vi "Device Scan SubVI.vi"(7 "Simulated Data":bool, 11 "error in (no error)":errorcluster) -> (3 "return count":u32, 4 "VISA INSTRUMENT 1":refnum<visa-resource-name>, 6 "VISA INSTRUMENT 2":refnum<visa-resource-name>, 8 "find list":string[](array[string]), 10 "Terminate":bool, 15 "error out":errorcluster)   [LabVIEW 2017]
uses:
  <vilib>/Instr/_visa.llb/VISA Find Search Mode.ctl
panel:
  # "This VI identifies the GPIB equipment attached to this computer, and searches to see it the following equipment\nis attached:\n\n(1)ASRL1::INSTR - Serial connection port between chromalox controller and computer\n(2)ASRL10::INSTR - Parallel connection port between elevator relays and computer"
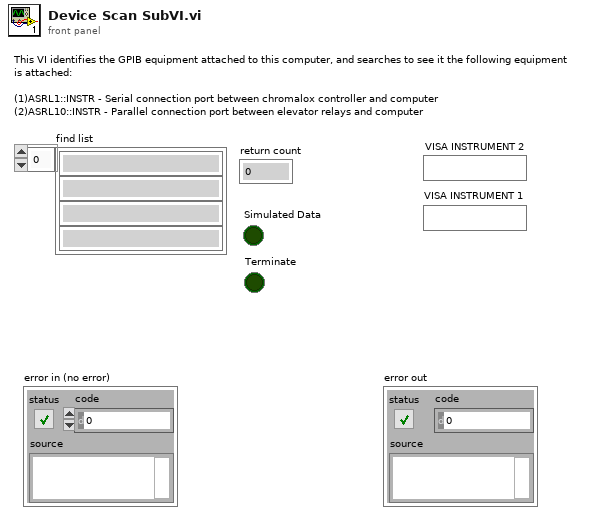
[diagram p1: front panel]
types:
  T1 = typedef "VISA Find Search Mode.ctl" = u32
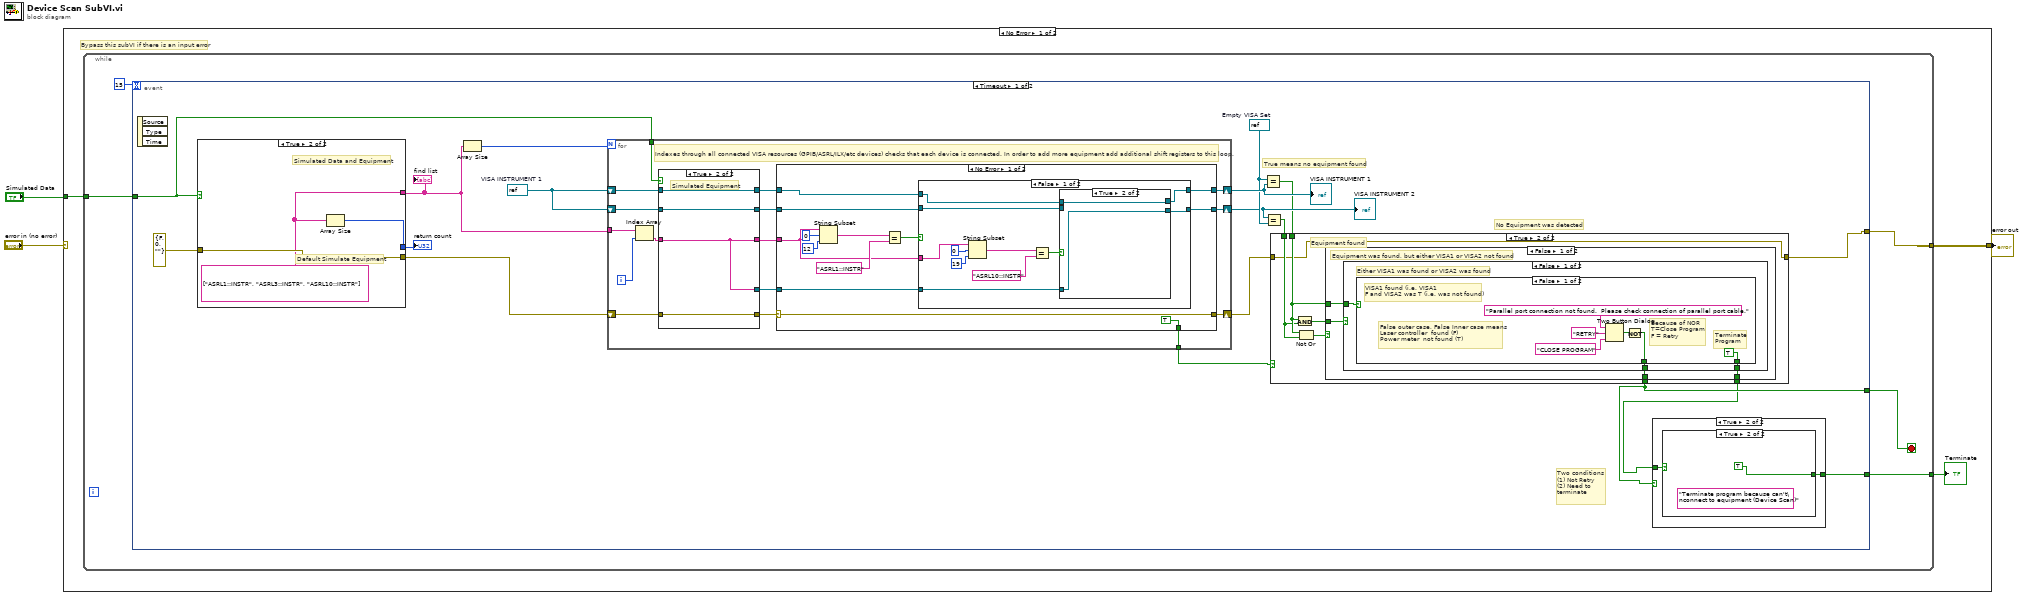
[diagram p0: block diagram]
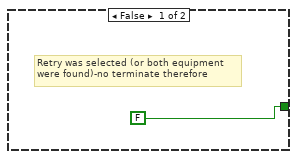
[diagram p2: hidden frame]
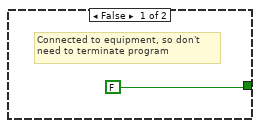
[diagram p3: hidden frame]
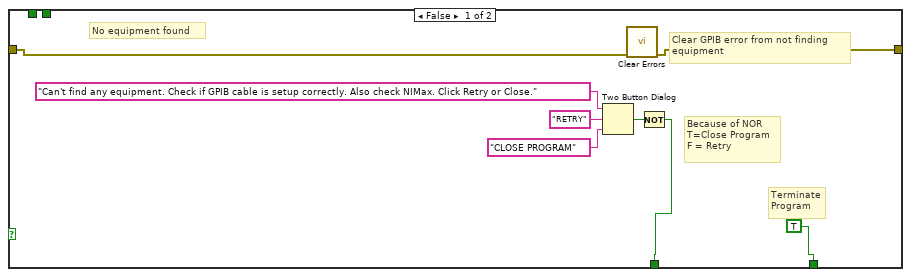
[diagram p4: hidden frame]
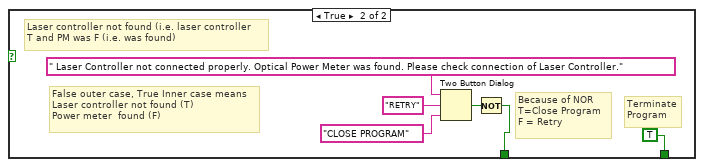
[diagram p5: hidden frame]
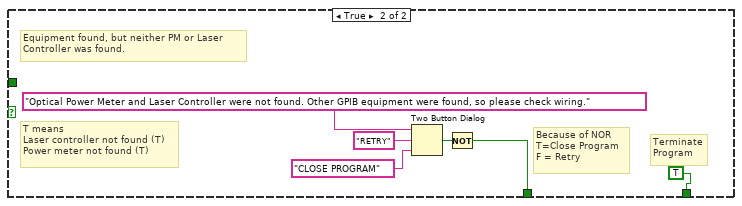
[diagram p6: hidden frame]
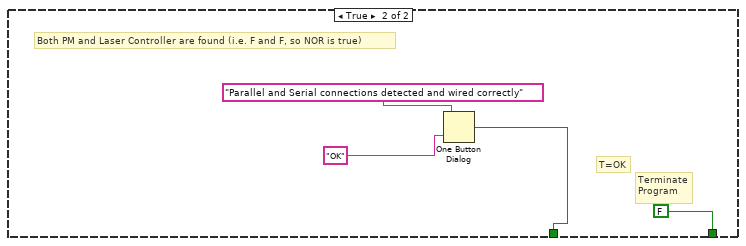
[diagram p7: hidden frame]
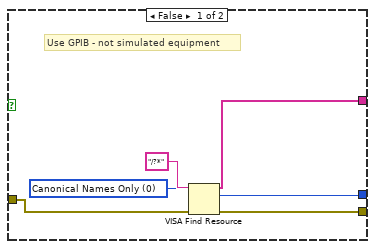
[diagram p8: hidden frame]
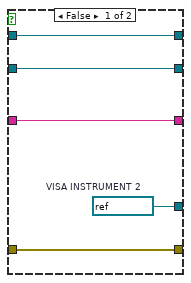
[diagram p9: hidden frame]
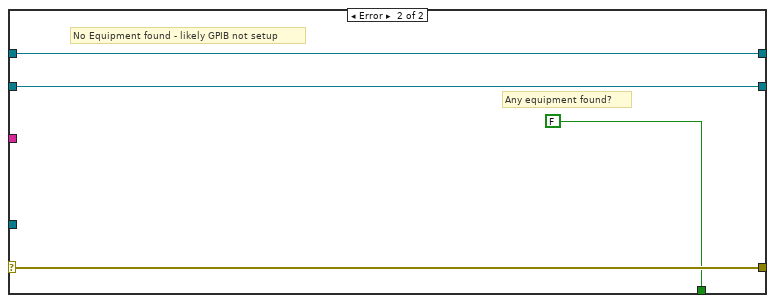
[diagram p12: hidden frame]
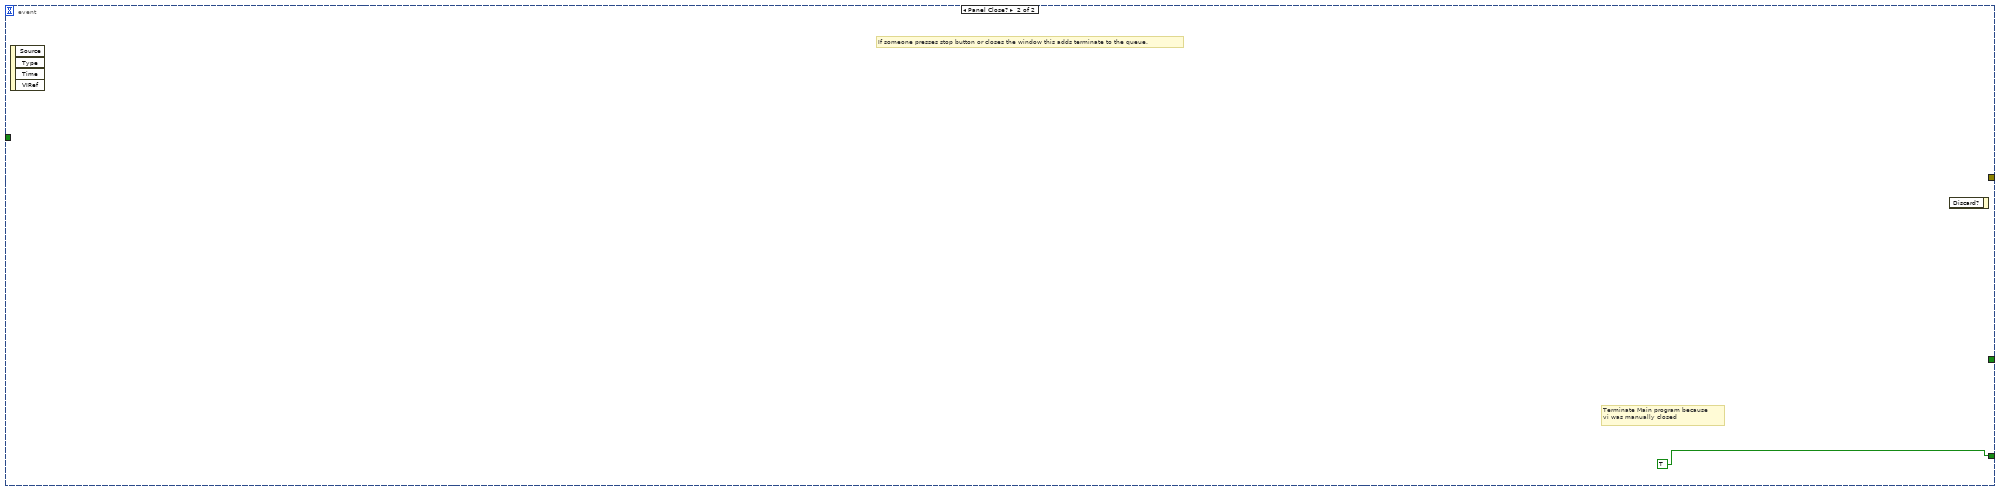
[diagram p13: hidden frame]
diagram:
  n1 = case shown="No Error" "error in (no error)" {
    selector: "error in (no error)" -> [_ w148]
    tunnel: [w6 w148] -> w2
    tunnel: "Simulated Data" -> [w5 _]
    frame No Error {
      # "Bypass this subVI if there is an input error"
      n2 = while {
        tunnel: [w10] -> w6
        tunnel: w5 -> [w9]
        tunnel: [w7] -> w4
        stop <- w11 stop-if-true
        n3 = event shown="[0] Timeout" {
          selector: _ -> [_ _]
          dyn-events: _ -> [_ _]
          timeout: 15 -> [_ _]
          tunnel: [w17 _] -> w11
          tunnel: [w13 _] -> w10
          tunnel: w9 -> [w21 _]
          tunnel: [w15 TRUE] -> w7
          event Timeout {
            w23 = refnum<visa-resource-name> refnum  # Empty VISA Set
            w12 = refnum<visa-resource-name> refnum  # VISA INSTRUMENT 1
            # "Two conditions\n(1) Not Retry\n(2) Need to\nterminate"
            # "No Equipment was detected"
            # "True means no equipment found"
            n4 = event-data() -> ()  [unwired: 1 in, 3 out]
            n5 = case shown="True" w21 {
              tunnel: [w84 w86] -> w28
              tunnel: [w81 w85] -> w27
              tunnel: [w80 w87] -> w26
              tunnel: errorcluster {"status"=FALSE, "code"=0, "source"=""} ("error in (no error) 2") -> [w79 w87]
              frame False {
                w82 = T1 0 items=["Canonical Names Only"=0, "Aliases Only"=2, "Include Matching Aliases"=3, "Include All Aliases"=4] ("Search Mode")
                # "Use GPIB - not simulated equipment"
                n6 = VISA Find Resource(8:w79, 10:w82, 11:"/?*" ("expression (\"?*\")")) -> (0:w80:errorcluster, 2:w84:u32, 3:w81:string[])
              }
              frame True {
                w85 = string[] ["ASRL1::INSTR", "ASRL3::INSTR", "ASRL10::INSTR"] ("Simulated Equipment List")
                # "Default Simulate Equipment"
                # "Simulated Data and Equipment"
                n7 = Array Size(array=w85) -> (size(s)=w86:i32)
              }
            }
            "find list" <- w27
            "return count" <- w28
            n8 = Array Size(array=w27) -> (size(s)=w29:i32)
            n9 = for {
              N: w29 -> [_]
              tunnel: w27 -> [w102]
              shift-right: [w97] -> w22
              shift-left: w12 -> [w93]
              shift-right: [w98] -> w24
              shift-left: w12 -> [w94]
              shift-right: [w95] -> w14
              shift-left: w26 -> [w99]
              tunnel: [w89] -> w18
              tunnel: w21 -> [w90]
              i -> [w103]
              # "Indexes through all connected VISA resources (GPIB/ASRL/ILX/etc devices) checks that each device is connected. In order to add more equipment add additional shift registers to this loop."
              n10 = Index Array(array=w102, index=w103) -> (element=w96:string)
              n11 = case shown="True" w90 {
                tunnel: [w106 w110] -> w101
                tunnel: [w105 w109] -> w100
                tunnel: w99 -> [w106 w110]
                tunnel: w96 -> [w105 w109]
                tunnel: w94 -> [w108 w112]
                tunnel: w93 -> [w107 w111]
                tunnel: [w108 w112] -> w92
                tunnel: [w107 w111] -> w91
                tunnel: [w104 w109] -> w88
                frame False {
                  w104 = refnum<visa-resource-name> refnum  # VISA INSTRUMENT 2
                }
                frame True {
                  # "Simulated Equipment"
                }
              }
              n12 = case shown="No Error" w101 {
                selector: w101 -> [w121 w146]
                tunnel: w100 -> [w117 _]
                tunnel: [w114 w143] -> w97
                tunnel: [w115 w144] -> w98
                tunnel: [w121 w146] -> w95
                tunnel: w91 -> [w120 w143]
                tunnel: w92 -> [w119 w144]
                tunnel: [TRUE FALSE] -> w89
                tunnel: w88 -> [w113 _]
                frame No Error {
                  n13 = String Subset(string=w117, offset (0)=0, length (rest)=12 ("length (rest)")) -> (substring=w118:string)
                  n14 = Equal?(x=w118, y="ASRL1::INSTR") -> (x = y?=w125:bool)
                  n15 = case shown="False" w125 {
                    tunnel: w120 -> [w129 w141]
                    tunnel: w119 -> [w130 w142]
                    tunnel: w117 -> [w132 _]
                    tunnel: [w126 w142] -> w115
                    tunnel: [w127 w141] -> w114
                    tunnel: w113 -> [w128 _]
                    frame False {
                      n16 = String Subset(string=w132, offset (0)=0, length (rest)=19 ("length (rest)")) -> (substring=w131:string)
                      n17 = Equal?(x=w131, y="ASRL10::INSTR") -> (x = y?=w135:bool)
                      n18 = case shown="True" w135 {
                        tunnel: w130 -> [w138 w140]
                        tunnel: w129 -> [w137 _]
                        tunnel: w128 -> [_ w139]
                        tunnel: [w138 w140] -> w126
                        tunnel: [w137 w139] -> w127
                        frame False {
                        }
                        frame True {
                        }
                      }
                    }
                    frame True {
                    }
                  }
                }
                frame Error {
                  # "Any equipment found?"
                  # "No Equipment found - likely GPIB not setup"
                }
              }
            }
            "VISA INSTRUMENT 1" <- w24
            "VISA INSTRUMENT 2" <- w22
            n19 = Equal?(x=w23, y=w24) -> (x = y?=w20:bool)
            n20 = Equal?(x=w22, y=w23) -> (x = y?=w19:bool)
            n21 = case shown="True" w18 {
              tunnel: [w38 w48] -> w17
              tunnel: w20 -> [_ w46]
              tunnel: w19 -> [_ w45]
              tunnel: [TRUE w44] -> w16
              tunnel: [w35 w43] -> w13
              tunnel: w14 -> [w36 w43]
              frame False {
                # "Clear GPIB error from not finding \nequipment"
                # "Terminate\nProgram"
                # "Because of NOR\nT=Close Program\nF = Retry"
                # "No equipment found"
                n22 = Two Button Dialog(message="Can't find any equipment. Check if GPIB cable is setup correctly. Also check NIMax. Click Retry or Close.", 1:"CLOSE PROGRAM", 2:"RETRY") -> (T button?=w42:bool)
                n23 = call <vilib>:"Clear Errors.vi"("error in (no error)"=w36) -> ("error out"=w35:errorcluster)  [unwired: 5 in, 1 out]
                n24 = Not(x=w42) -> (.not. x?=w38:bool)
              }
              frame True {
                # "Equipment found"
                n25 = And(x=w46, y=w45) -> (x .and. y?=w49:bool)
                n26 = Not Or(1:w45, 2:w46) -> (0:w47:bool)
                n27 = case shown="False" w47 {
                  tunnel: w49 -> [w53 _]
                  tunnel: [w52 w77] -> w48
                  tunnel: w46 -> [w51 _]
                  tunnel: [w50 FALSE] -> w44
                  frame False {
                    # "Equipment was found, but either VISA1 or VISA2 not found"
                    n28 = case shown="False" w53 {
                      tunnel: [w55 w70] -> w52
                      tunnel: w51 -> [w56 _]
                      tunnel: [w54 TRUE] -> w50
                      frame False {
                        # "Either VISA1 was found or VISA2 was found"
                        n29 = case shown="False" w56 {
                          tunnel: [w58 w64] -> w55
                          tunnel: [TRUE TRUE] -> w54
                          frame False {
                            # "Terminate\nProgram"
                            # "False outer case, False Inner case means\nLaser controller  found (F)\nPower meter  not found (T)"
                            # "Because of NOR\nT=Close Program\nF = Retry"
                            # "VISA1 found (i.e. VISA1\nF and VISA2 was T (i.e. was not found)"
                            n30 = Two Button Dialog(message="Parallel port connection not found.  Please check connection of parallel port cable.", 1:"CLOSE PROGRAM", 2:"RETRY") -> (T button?=w59:bool)
                            n31 = Not(x=w59) -> (.not. x?=w58:bool)
                          }
                          frame True {
                            # "Terminate\nProgram"
                            # "False outer case, True Inner case means\nLaser controller not found (T)\nPower meter  found (F)"
                            # "Because of NOR\nT=Close Program\nF = Retry"
                            # "Laser controller not found (i.e. laser controller\nT and PM was F (i.e. was found)"
                            n32 = Two Button Dialog(message=" Laser Controller not connected properly. Optical Power Meter was found. Please check connection of Laser Controller.", 1:"CLOSE PROGRAM", 2:"RETRY") -> (T button?=w65:bool)
                            n33 = Not(x=w65) -> (.not. x?=w64:bool)
                          }
                        }
                      }
                      frame True {
                        # "Terminate\nProgram"
                        # "T means\nLaser controller not found (T)\nPower meter not found (T)"
                        # "Because of NOR\nT=Close Program\nF = Retry"
                        # "Equipment found, but neither PM or Laser\nController was found."
                        n34 = Two Button Dialog(message="Optical Power Meter and Laser Controller were not found. Other GPIB equipment were found, so please check wiring.", 1:"CLOSE PROGRAM", 2:"RETRY") -> (T button?=w71:bool)
                        n35 = Not(x=w71) -> (.not. x?=w70:bool)
                      }
                    }
                  }
                  frame True {
                    # "Terminate\nProgram"
                    # "T=OK"
                    # "Both PM and Laser Controller are found (i.e. F and F, so NOR is true)"
                    n36 = One Button Dialog(message="Parallel and Serial connections detected and wired correctly", button name ("OK")="OK") -> (true=w77:bool)
                  }
                }
              }
            }
            n37 = case shown="True" w17 {
              tunnel: w16 -> [_ w32]
              tunnel: [FALSE w31] -> w15
              frame False {
                # "Retry was selected (or both equipment\nwere found)-no terminate therefore"
              }
              frame True {
                n38 = case shown="True" w32 {
                  tunnel: [FALSE TRUE] -> w31
                  frame False {
                    # "Connected to equipment, so don't\nneed to terminate program"
                  }
                  frame True {
                    (unwired) "Terminate program because can't\nconnect to equipment (Device Scan)"
                  }
                }
              }
            }
          }
          event Panel Close? {
            # "Terminate Main program because \nvi was manually closed"
            # "If someone presses stop button or closes the window this adds terminate to the queue."
            n39 = event-data() -> ()  [unwired: 1 in, 4 out]
            n40 = event-data() -> ()  [unwired: 2 in, 1 out]
          }
        }
      }
      "Terminate" <- w4
    }
    frame Error {
      # "Bypass this subvi if error."
    }
  }
  "error out" <- w2
